vi "maszynas stanow do arduino.vi"() -> ()   [LabVIEW 2025]
doc: "Use this template to build a standard state machine design pattern. Each state executes code and determines which state to transition to. Contrast this design pattern with the User Interface Event Handler pattern, in which code executes in response to user actions. Contrast this design pattern also with the Queued Message Handler pattern, in which each message handling code can queue zero or more new messages.\nNote: This template does not contain the most recent programming guidelines recommended by National Instruments. For a complete, project-based implementation of the Standard State Machine pattern, use the Create Project dialog box instead of this template."
uses:
  maszyna stanow do arduino.ctl
  <vilib>/MakerHub/LINX/LMH-LINX.lvlib
  <vilib>/MakerHub/LINX/Public/Peripherals/Digital/Digital Read 1 Chan.vi
  <vilib>/MakerHub/LINX/Public/Sensors/Motion/Servo/Servo.lvlib
  <vilib>/MakerHub/LINX/Public/Utilities/Open Serial.vi
  <vilib>/MakerHub/LINX/Public/Sensors/Motion/Servo/Servo Open N Channels.vi
  <vilib>/MakerHub/LINX/Public/Sensors/Motion/Servo/Servo Close N Channels.vi
  <vilib>/MakerHub/LINX/Public/Sensors/Motion/Servo/Servo Set Pulse Width N Channels.vi
  <vilib>/MakerHub/LINX/Public/Peripherals/Digital/Digital Read N Chans.vi
  <vilib>/MakerHub/LINX/Public/Peripherals/Digital/Digital Write N Chans.vi
  <vilib>/MakerHub/LINX/Private/Type Defs/LINX Ref.ctl
  <vilib>/MakerHub/LINX/Private/Type Defs/Platform.ctl
  <vilib>/MakerHub/LINX/Private/Type Defs/Interface.ctl
  <vilib>/MakerHub/LINX/Private/Device/Type Defs/LINX Device Config.ctl
  <vilib>/MakerHub/LINX/Private/Device/Device.lvlib
  <vilib>/MakerHub/LINX/Private/Device/Type Defs/TCP Config.ctl
  <vilib>/MakerHub/LINX/Private/Device/Type Defs/Channels.ctl
panel:
  in  "DI Channels":u8[](array[numeric])
  in  "Servo Channels":u8[](array[numeric])
  in  "Sterowanie z przycisków":bool
  in  "Sterowanie z Pythona":bool
  in  "LINX Resource 2":T1
  in  "LINX Resource":T1
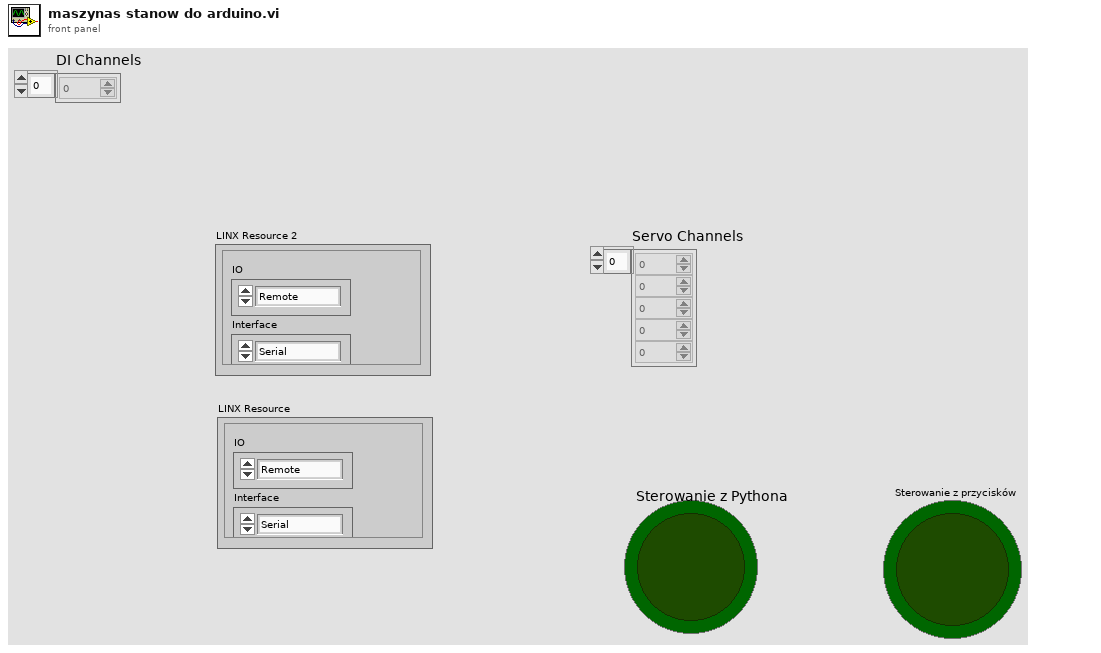
[diagram p1: front panel]
types:
  T1 = typedef "LMH-LINX.lvlib/LINX Ref.ctl" = cluster{"IO":T2, "Interface":T3, "LINX Device Config":T4}
  T2 = typedef "LMH-LINX.lvlib/Platform.ctl" = enum16{"Remote", "Local"}
  T3 = typedef "LMH-LINX.lvlib/Interface.ctl" = enum16{"Serial", "TCP"}
  T4 = typedef "LMH-LINX.lvlib/Device.lvlib/LINX Device Config.ctl" = cluster{"Interface":T3, "COM Port":refnum<visa-resource-name>, "TCP Configuration":T5, "Device Family":u8, "Device ID":u8, "Device Name":string, "TCP Ref":refnum<k5>, "Channels":T6}
  T5 = typedef "LMH-LINX.lvlib/Device.lvlib/TCP Config.ctl" = cluster{"IP Address":string, "Port":u16}
  T6 = typedef "LMH-LINX.lvlib/Channels.ctl" = cluster{"DI":u8[], "DO":u8[], "AI":u8[], "AO":u8[], "PWM":u8[], "QE":u8[], "UART":u8[], "I2C 2":u8[], "SPI":u8[], "CAN":u8[], "Servo":u8[], "AI Ref (V)":dbl, "AI Resolution (Bits)":u8, "AO Ref (V)":dbl, "AO Resolution (Bits)":u8}
  T7 = typedef "maszyna stanow do arduino.ctl" = enum16{"Choose mode", "Set by buttons", "Set by py", "Initialize", "Stop"}
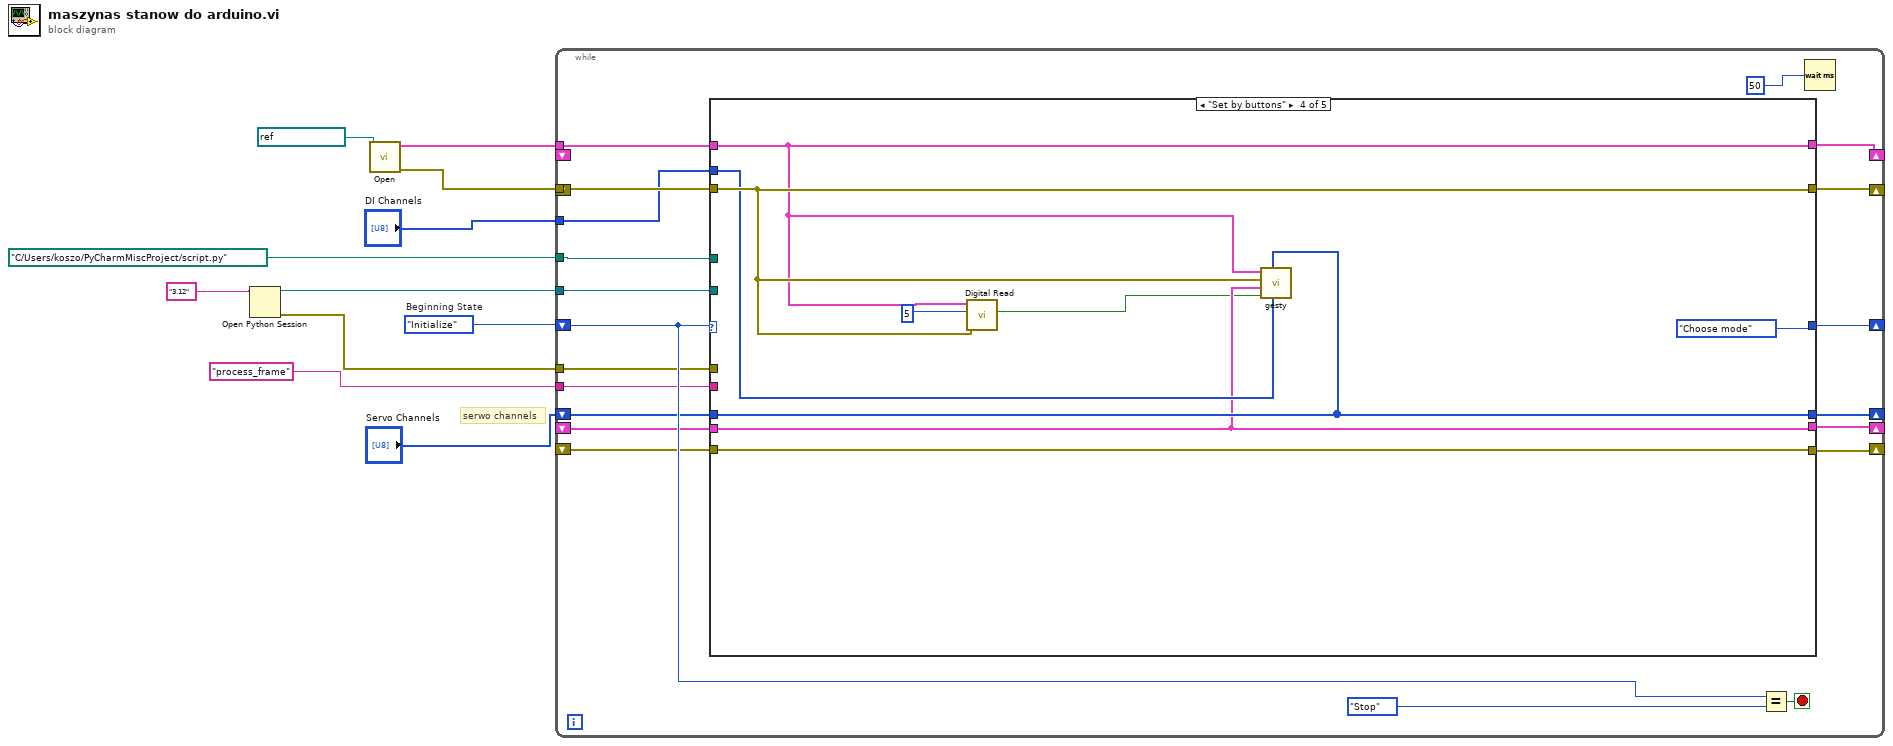
[diagram p0: block diagram]
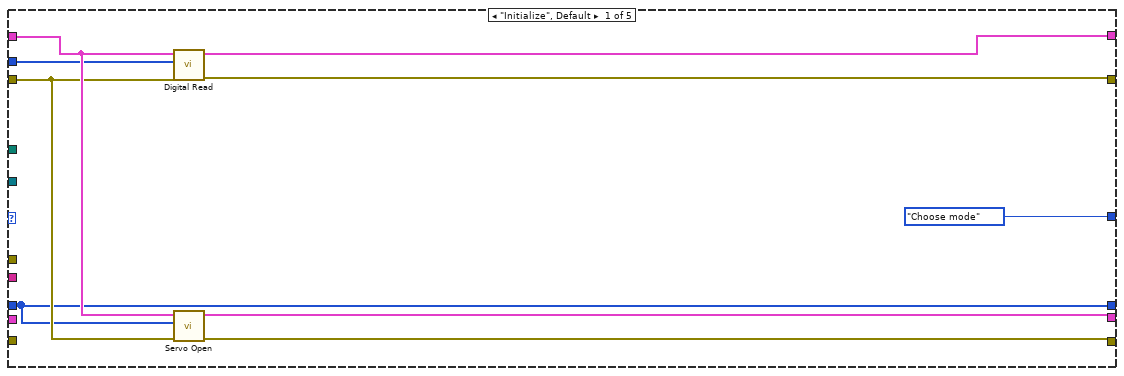
[diagram p2: hidden frame]
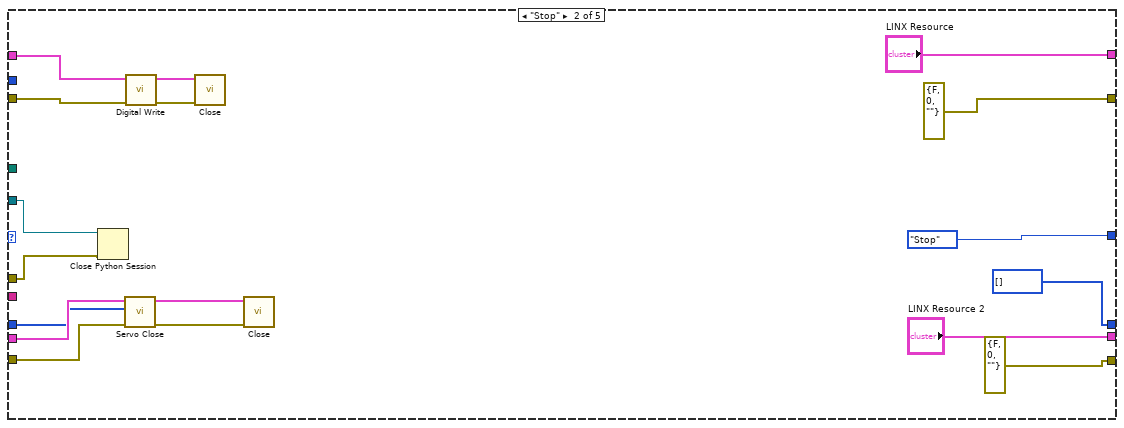
[diagram p3: hidden frame]
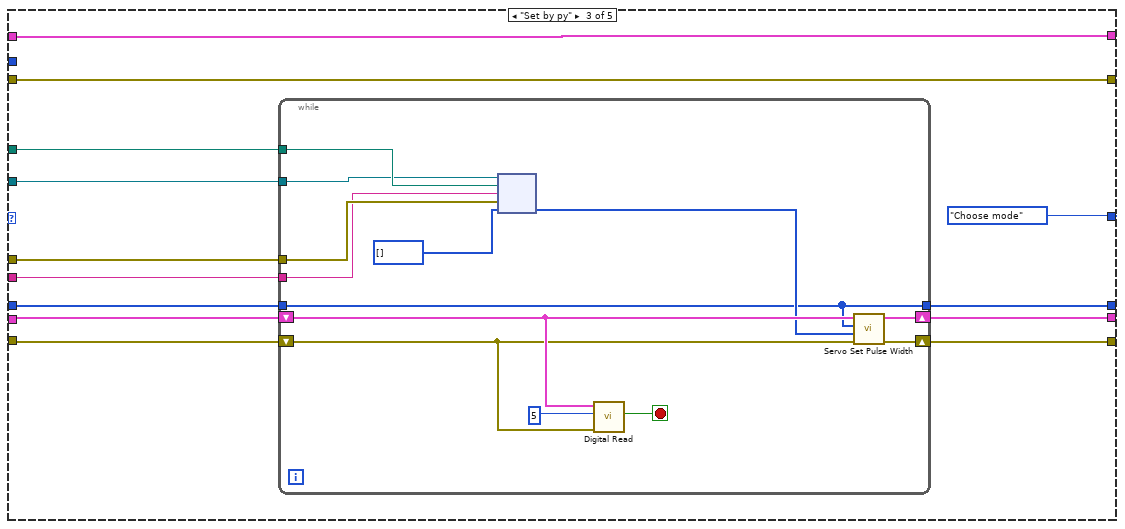
[diagram p4: hidden frame]
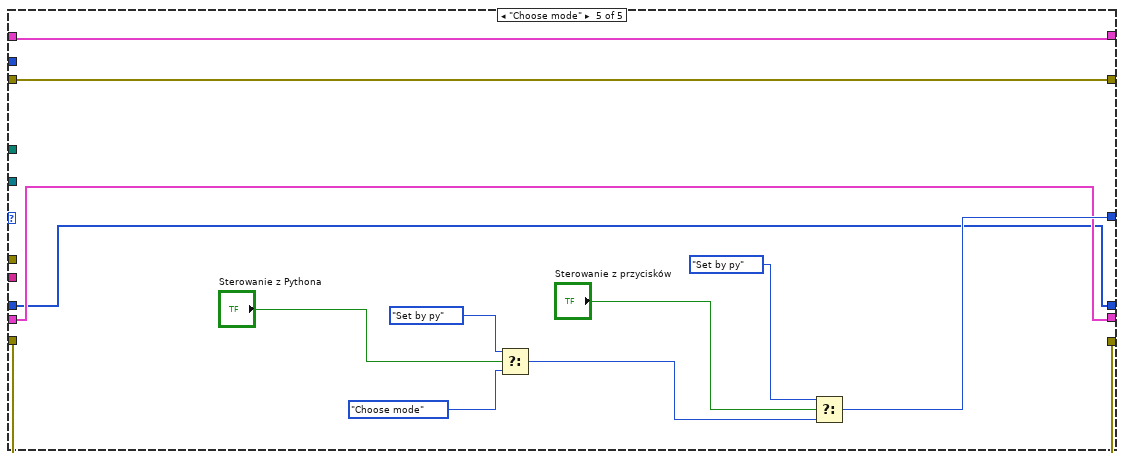
[diagram p5: hidden frame]
diagram:
  w11 = maszyna_stanow_do_arduino."Initialize"  # Beginning State
  # "serwo channels"
  n1 = Open Python Session(python version="3.12" ("Python version")) -> (session out=w5:refnum<k35>, error out=w4:errorcluster)  [unwired: 2 in]
  n2 = call-poly <vilib>:"Open.vi"("Serial Port"=refnum<visa-resource-name> "COM5") -> ("Error Out"=w8:errorcluster, "LINX Resource"=w9:T1)  [unwired: 8 in, 1 out]
  n3 = while {
    shift-right: [w29] -> _
    shift-left: w11 -> [w23]
    tunnel: w9 -> [w27]
    tunnel: w8 -> [w26]
    shift-right: [w25] -> _
    shift-left: _ -> [_]
    shift-right: [w24] -> _
    shift-left: _ -> [_]
    shift-right: [w13] -> _
    shift-left: "Servo Channels" -> [w14]
    shift-right: [w22] -> _
    shift-left: _ -> [w20]
    shift-right: [w21] -> _
    shift-left: _ -> [w19]
    tunnel: path "C:/Users/koszo/PyCharmMiscProject/script.py" ("module path") -> [w18]
    tunnel: w5 -> [w17]
    tunnel: w4 -> [w16]
    tunnel: "process_frame" ("function name") -> [w15]
    tunnel: "DI Channels" -> [w12]
    stop <- w31 stop-if-true
    n4 = case shown="\"Set by buttons\"" w23 {
      tunnel: [maszyna_stanow_do_arduino."Choose mode" ("States") maszyna_stanow_do_arduino."Stop" ("Next State") maszyna_stanow_do_arduino."Choose mode" ("States") maszyna_stanow_do_arduino."Choose mode" ("States") w98] -> w29
      tunnel: w27 -> [w36 w54 w68 w85 w97]
      tunnel: w26 -> [w35 w52 w67 w88 w96]
      tunnel: [w40 "LINX Resource" w68 w85 w97] -> w25
      tunnel: [w39 errorcluster {"status"=FALSE, "code"=0, "source"=""} ("Error Out") w67 w88 w96] -> w24
      tunnel: [w38 "LINX Resource 2" w70 w86 w95] -> w22
      tunnel: [w37 errorcluster {"status"=FALSE, "code"=0, "source"=""} ("Error Out") w69 w91 w94] -> w21
      tunnel: w20 -> [_ w47 w65 w86 w95]
      tunnel: w19 -> [_ w48 w64 w91 w94]
      tunnel: w18 -> [_ _ w63 _ _]
      tunnel: w17 -> [_ w43 w62 _ _]
      tunnel: w16 -> [_ w44 w61 _ _]
      tunnel: w15 -> [_ _ w60 _ _]
      tunnel: w14 -> [w33 w42 w59 w89 w93]
      tunnel: [w33 u8[] [] ("Servo Channels") w58 w89 w93] -> w13
      tunnel: w12 -> [w32 _ _ w87 _]
      frame "Initialize", Default {
        n5 = call-poly <vilib>:"Digital Read.vi"("Error In"=w35, "DI Channels"=w32, "LINX Resource"=w36) -> ("Error Out"=w39:errorcluster, "LINX Resource"=w40:T1)  [unwired: 6 in, 1 out]
        n6 = call-poly <vilib>:"Servo Open.vi"("Error In"=w35, "Servo Channels"=w33, "LINX Resource"=w36) -> ("Error Out"=w37:errorcluster, "LINX Resource"=w38:T1)  [unwired: 7 in]
      }
      frame "Stop" {
        n7 = Close Python Session(session in=w43, error in=w44) -> ()  [unwired: 1 out]
        n8 = call-poly <vilib>:"Servo Close.vi"("Error In"=w48, "Servo Channels"=w42, "LINX Resource"=w47) -> ("Error Out"=w49:errorcluster, "LINX Resource"=w50:T1)  [unwired: 7 in]
        n9 = call-poly <vilib>:"Digital Write.vi"("Error In"=w52, "LINX Resource"=w54) -> ("Error Out"=w51:errorcluster, "LINX Resource"=w53:T1)  [unwired: 8 in]
        n10 = call <vilib>:"Close.vi"("Error In"=w51, "LINX Resource"=w53) -> ()  [unwired: 9 in, 1 out]
        n11 = call <vilib>:"Close.vi"("Error In"=w49, "LINX Resource"=w50) -> ()  [unwired: 9 in, 1 out]
      }
      frame "Set by py" {
        n12 = while {
          shift-right: [w83] -> w70
          shift-left: w65 -> [w79]
          shift-right: [w82] -> w69
          shift-left: w64 -> [w78]
          tunnel: w63 -> [w77]
          tunnel: w62 -> [w76]
          tunnel: w61 -> [w75]
          tunnel: w60 -> [w74]
          tunnel: w59 -> [w71]
          tunnel: [w71] -> w58
          stop <- w80 stop-if-true
          n13 = node(w76, w77, w74, w75, u16[] []) -> (w72:u16[])  [unwired: 4 out]
          n14 = call-poly <vilib>:"Digital Read.vi"("Error In"=w78, "DI Channel"=u8 5, "LINX Resource"=w79) -> ("DI Value"=w80:bool)  [unwired: 6 in, 2 out]
          n15 = call-poly <vilib>:"Servo Set Pulse Width.vi"("Error In"=w78, "Pulse Widths (uS)"=w72, "Servo Channels"=w71, "LINX Resource"=w79) -> ("Error Out"=w82:errorcluster, "LINX Resource"=w83:T1)  [unwired: 6 in]
        }
      }
      frame "Set by buttons" {
        n16 = call-poly <vilib>:"Digital Read.vi"("Error In"=w88, "DI Channel"=u8 5, "LINX Resource"=w85) -> ("DI Value"=w84:bool)  [unwired: 6 in, 2 out]
        n17 = call "gesty.vi"("Przyciski"=w87, "Kanały serwa"=w89, "zatrzymanie wybierania gestów"=w84, "LINX SERWO"=w86, "Error In"=w88, "DIGITAL READ"=w85) -> ()  [unwired: 6 in]
      }
      frame "Choose mode" {
        n18 = Select(t=maszyna_stanow_do_arduino."Set by py" ("States"), s="Sterowanie z Pythona", f=maszyna_stanow_do_arduino."Choose mode" ("States")) -> (s? t:f=w100:T7)
        n19 = Select(t=maszyna_stanow_do_arduino."Set by py" ("States"), s="Sterowanie z przycisków", f=w100) -> (s? t:f=w98:T7)
      }
    }
    n20 = Equal?(x=w23, y=maszyna_stanow_do_arduino."Stop" ("States")) -> (x = y?=w31:bool)
    n21 = Wait (ms)(milliseconds to wait=u32 50) -> ()  [unwired: 1 out]
  }
